vi "keyboard_control_drone.vi"(0 "Take/off":refnum<vi>, 5 "NavData Out 2":T1, 9 "resulting string":string, 11 "Move Ammount":dbl=0.6, 12 "Auto_mode":refnum<vi>) -> (4 "Cluster":cluster{i32, i32, i32, i32}, 6 "Hover":bool)   [LabVIEW 2015]
uses:
  <vilib>/LVH/AR Drone Toolkit/Decode NavData/Typedefs/NavData Demo.ctl
  video_global.vi
  <vilib>/LVH/AR Drone Toolkit/AR Drone.lvlib
panel:
  out "height_speed":dbl
  out "resulting string 2":string
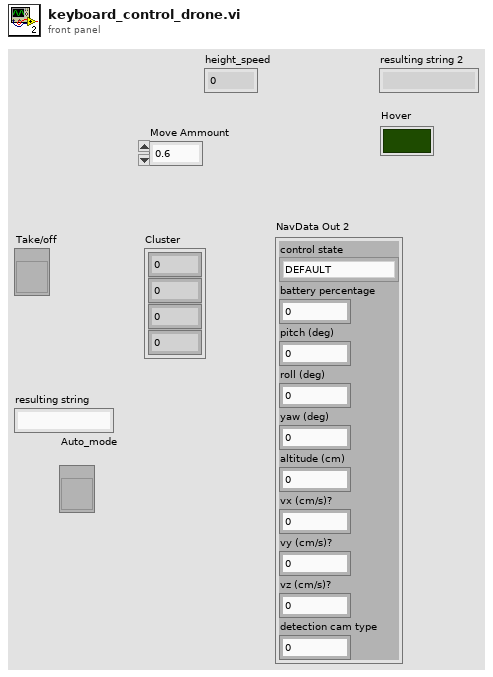
[diagram p1: front panel]
types:
  T1 = typedef "AR Drone.lvlib/NavData Demo.ctl" = cluster{"control state":enum32{"DEFAULT", "INIT", "LANDING", "FLYING", "HOVERING", "TEST", "TRANS_TAKEOFF", "TRANS_GOTOFIX", "TRANS_LANDING"}, "battery percentage":u32, "pitch (deg)":sgl, "roll (deg)":sgl, "yaw (deg)":sgl, "altitude (cm)":u32, "vx (cm/s)?":sgl, "vy (cm/s)?":sgl, "vz (cm/s)?":sgl, "detection cam type":u32}
  T2 = cluster{"Move Ammount":dbl, "Move Ammount":dbl, "Move Ammount":dbl, "Move Ammount":dbl}
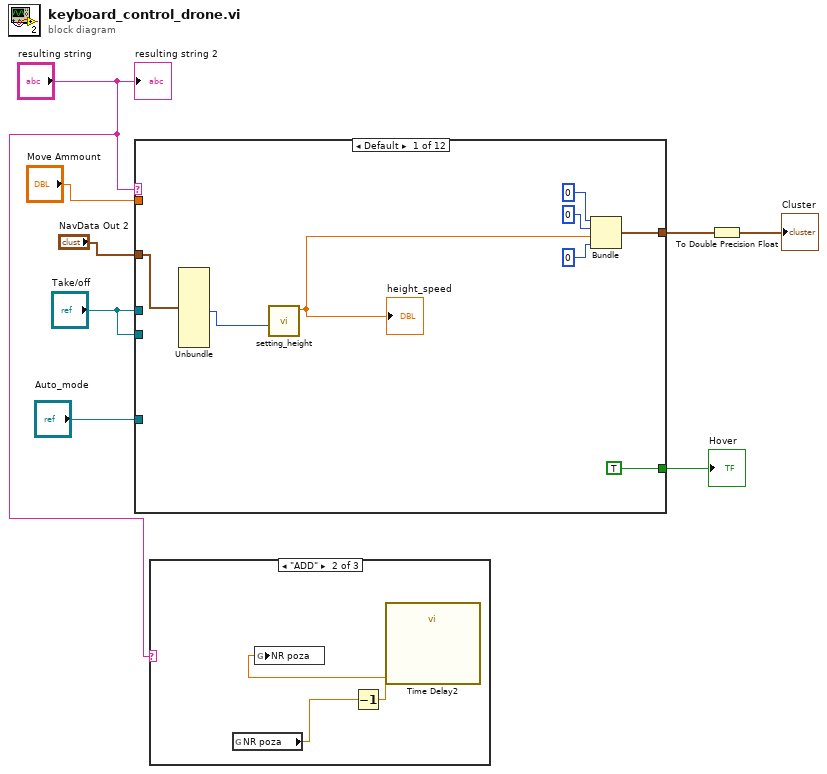
[diagram p0: block diagram]
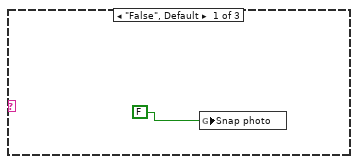
[diagram p2: hidden frame]
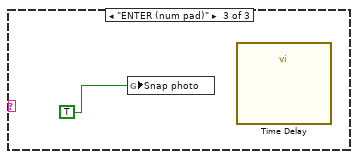
[diagram p3: hidden frame]
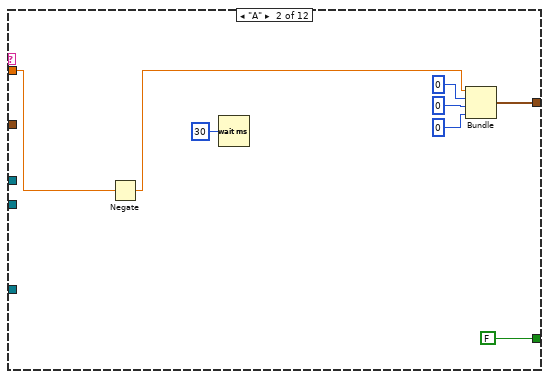
[diagram p4: hidden frame]
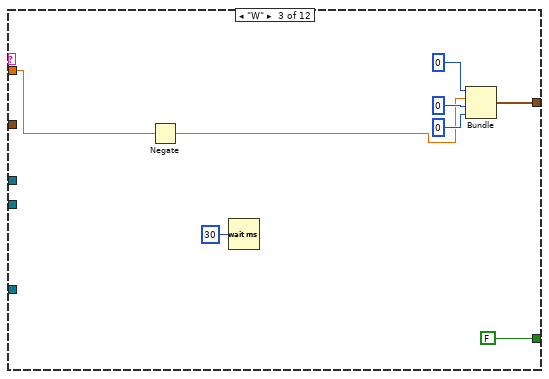
[diagram p5: hidden frame]
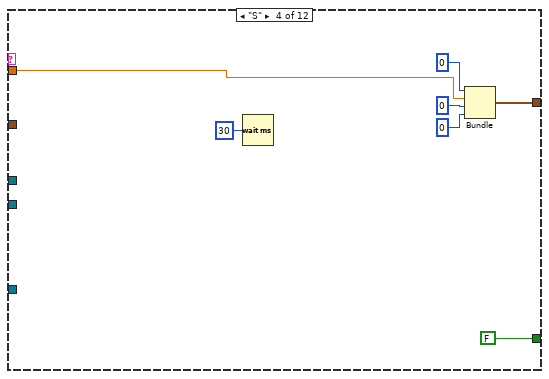
[diagram p6: hidden frame]
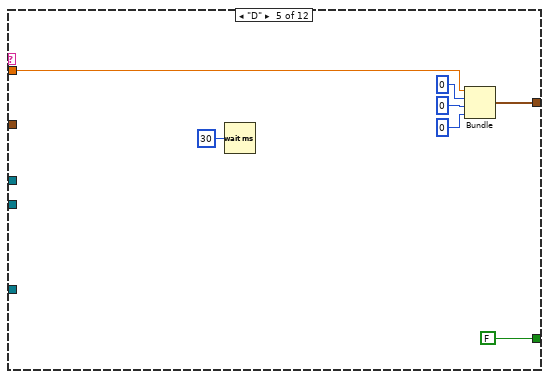
[diagram p7: hidden frame]
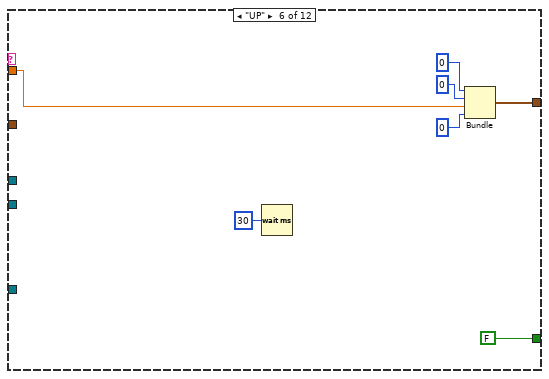
[diagram p8: hidden frame]
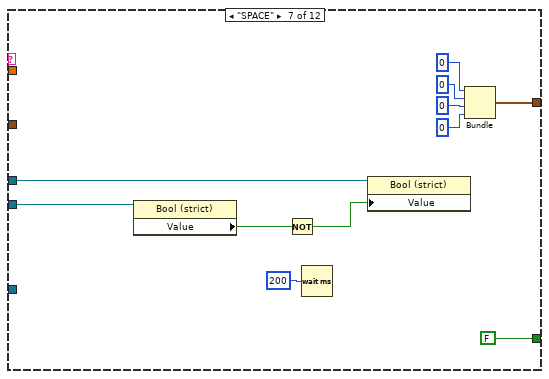
[diagram p9: hidden frame]
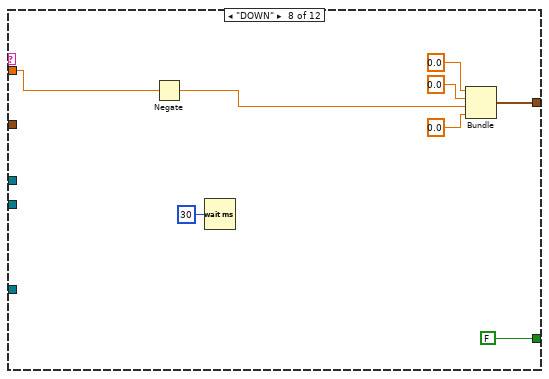
[diagram p10: hidden frame]
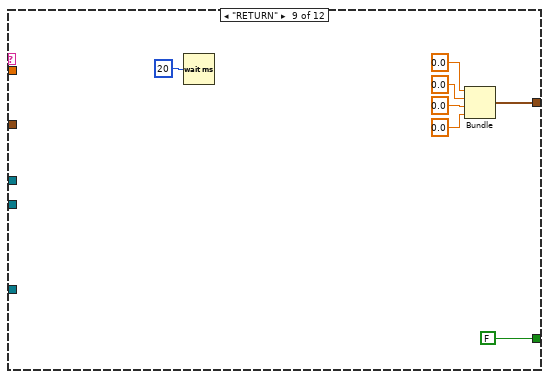
[diagram p11: hidden frame]
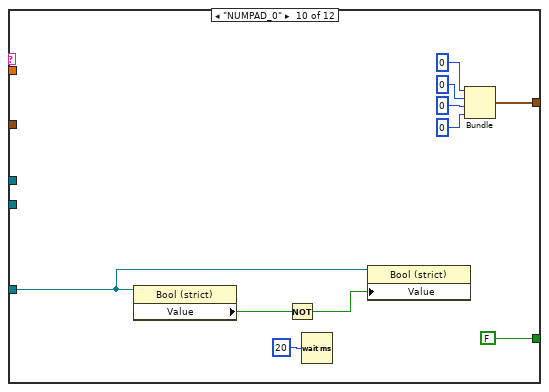
[diagram p12: hidden frame]
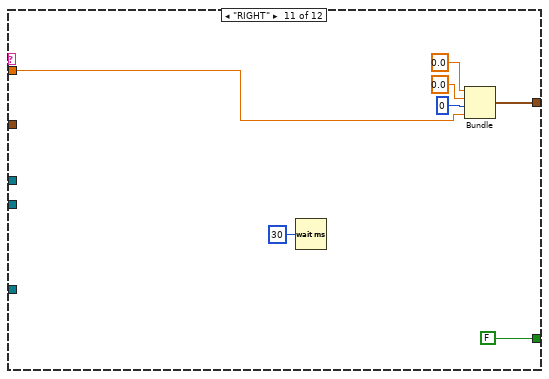
[diagram p13: hidden frame]
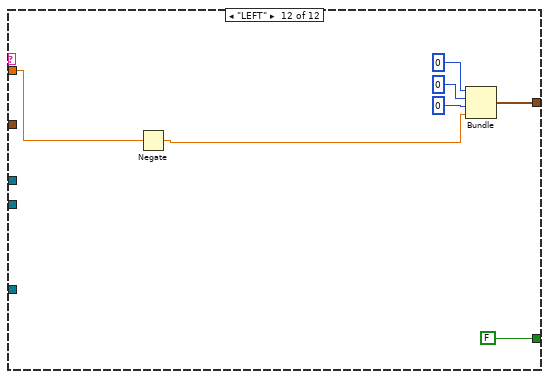
[diagram p14: hidden frame]
diagram:
  n1 = case shown="Default" "resulting string" {
    tunnel: [w13 w21 w29 w36 w43 w50 w60 w69 w75 w82 w93 w100] -> w7
    tunnel: "Take/off" -> [_ _ _ _ _ _ w57 _ _ _ _ _]
    tunnel: "Take/off" -> [_ _ _ _ _ _ w56 _ _ _ _ _]
    tunnel: "Auto_mode" -> [_ _ _ _ _ _ _ _ _ w88 _ _]
    tunnel: [TRUE FALSE FALSE FALSE FALSE FALSE FALSE FALSE FALSE FALSE FALSE FALSE] -> w4
    tunnel: "NavData Out 2" -> [w11 _ _ _ _ _ _ _ _ _ _ _]
    tunnel: "Move Ammount" -> [_ w19 w27 w34 w41 w48 _ w67 _ _ w91 w98]
    frame Default {
      n2 = Unbundle(w11) -> ("altitude (cm)"=w10:u32)  [unwired: 9 out]
      n3 = call "setting_height.vi"("Current_height"=w10) -> ("height_speed"=w9:dbl)  [unwired: 10 in]
      "height_speed" <- w9
      n4 = Bundle(0, 0, "height_speed"=w9, 0) -> (w13:cluster{i32, i32, "height_speed":dbl, i32})  [unwired: 1 in]
    }
    frame "A" {
      n5 = Negate(x=w19) -> (-x=w18:dbl)
      n6 = Wait (ms)(milliseconds to wait=u32 30) -> ()  [unwired: 1 out]
      n7 = Bundle(w18, 0, 0, 0) -> (w21:cluster{dbl, i32, i32, i32})  [unwired: 1 in]
    }
    frame "W" {
      n8 = Negate(x=w27) -> (-x=w26:dbl)
      n9 = Wait (ms)(milliseconds to wait=u32 30) -> ()  [unwired: 1 out]
      n10 = Bundle(0, w26, 0, 0) -> (w29:cluster{i32, dbl, i32, i32})  [unwired: 1 in]
    }
    frame "S" {
      n11 = Wait (ms)(milliseconds to wait=u32 30) -> ()  [unwired: 1 out]
      n12 = Bundle(0, "Move Ammount"=w34, 0, 0) -> (w36:cluster{i32, "Move Ammount":dbl, i32, i32})  [unwired: 1 in]
    }
    frame "D" {
      n13 = Wait (ms)(milliseconds to wait=u32 30) -> ()  [unwired: 1 out]
      n14 = Bundle("Move Ammount"=w41, 0, 0, 0) -> (w43:cluster{"Move Ammount":dbl, i32, i32, i32})  [unwired: 1 in]
    }
    frame "UP" {
      n15 = Wait (ms)(milliseconds to wait=u32 30) -> ()  [unwired: 1 out]
      n16 = Bundle(0, 0, "Move Ammount"=w48, 0) -> (w50:cluster{i32, i32, "Move Ammount":dbl, i32})  [unwired: 1 in]
    }
    frame "SPACE" {
      n17 = property class="Bool (strict)"(reference=w56) -> ("Value"=w59:bool)  [unwired: 1 in, 2 out]
      n18 = Not(x=w59) -> (.not. x?=w58:bool)
      n19 = Wait (ms)(milliseconds to wait=u32 200) -> ()  [unwired: 1 out]
      n20 = property class="Bool (strict)"(reference=w57, "Value"=w58) -> ()  [unwired: 1 in, 2 out]
      n21 = Bundle(0, 0, 0, 0) -> (w60:cluster{i32, i32, i32, i32})  [unwired: 1 in]
    }
    frame "DOWN" {
      n22 = Negate(x=w67) -> (-x=w66:dbl)
      n23 = Wait (ms)(milliseconds to wait=u32 30) -> ()  [unwired: 1 out]
      n24 = Bundle(0.0, 0.0, w66, 0.0) -> (w69:cluster{dbl, dbl, dbl, dbl})  [unwired: 1 in]
    }
    frame "RETURN" {
      n25 = Wait (ms)(milliseconds to wait=u32 20) -> ()  [unwired: 1 out]
      n26 = Bundle(0.0, 0.0, 0.0, 0.0) -> (w75:cluster{dbl, dbl, dbl, dbl})  [unwired: 1 in]
    }
    frame "NUMPAD_0" {
      n27 = property class="Bool (strict)"(reference=w88) -> ("Value"=w89:bool)  [unwired: 1 in, 2 out]
      n28 = Not(x=w89) -> (.not. x?=w87:bool)
      n29 = Wait (ms)(milliseconds to wait=u32 20) -> ()  [unwired: 1 out]
      n30 = property class="Bool (strict)"(reference=w88, "Value"=w87) -> ()  [unwired: 1 in, 2 out]
      n31 = Bundle(0, 0, 0, 0) -> (w82:cluster{i32, i32, i32, i32})  [unwired: 1 in]
    }
    frame "RIGHT" {
      n32 = Wait (ms)(milliseconds to wait=u32 30) -> ()  [unwired: 1 out]
      n33 = Bundle(0.0, 0.0, 0, "Move Ammount"=w91) -> (w93:cluster{dbl, dbl, i32, "Move Ammount":dbl})  [unwired: 1 in]
    }
    frame "LEFT" {
      n34 = Negate(x=w98) -> (-x=w97:dbl)
      n35 = Bundle(0, 0, 0, w97) -> (w100:cluster{i32, i32, i32, dbl})  [unwired: 1 in]
    }
  }
  "Hover" <- w4
  n36 = case shown="\"ADD\"" "resulting string" {
    frame "False", Default {
      n37 = global write "video_global.vi" "Snap photo"(FALSE) -> ()
    }
    frame "ADD" {
      n38 = global read "video_global.vi" "NR poza"() -> (w106:dbl)
      n39 = Decrement(x=w106) -> (x-1=w105:dbl)
      n40 = global write "video_global.vi" "NR poza"(w105) -> ()
      n41 = call "Time Delay2"() -> ()  [unwired: 11 in, 1 out]
    }
    frame "ENTER (num pad)" {
      n42 = global write "video_global.vi" "Snap photo"(TRUE) -> ()
      n43 = call "Time Delay"() -> ()  [unwired: 11 in, 1 out]
    }
  }
  n44 = To Double Precision Float(number=w7) -> (double precision float=→"Cluster":T2)
  "resulting string 2" <- "resulting string"
